vi "Msg To Self.vi"(9 "Priority Msg?":bool, 10 "Msg":refnum<class "Msg Strategy.lvclass">, 11 "Self Actor in":refnum<class "Self Actor.lvclass">) -> (0 "error out":errorcluster)   [LabVIEW 2021, in "LVCAM.lvlib" / "Self Actor.lvclass"]
uses:
  Self Actor.lvclass
  Msg Strategy/Msg Strategy.lvclass
  Self Actor.lvclass/Self Actor.ctl
  LVCAM.lvlib
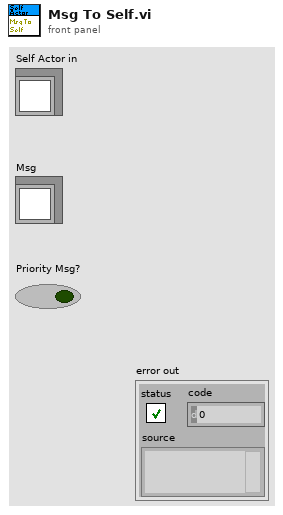
[diagram p1: front panel]
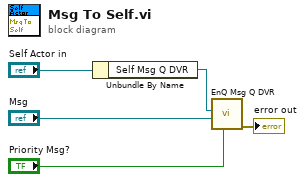
[diagram p0: block diagram]
diagram:
  n1 = Unbundle By Name("Self Actor in") -> ("Self Msg Q DVR"=w5:refnum<data-value>)
  n2 = call "EnQ Msg Q DVR.vi"("Priority Msg?"="Priority Msg?", "Msg"="Msg", "Msg Q DVR"=w5) -> ("error out"=→"error out":errorcluster)  [unwired: 8 in]
